vi "Wait Event.vi"(7 "Keep Event Reg (F)":bool, 8 "error in (no error)":errorcluster, 9 "Timeout mS (-1)":i32=-1, 11 "Future in":refnum<class "Future.lvclass">) -> (0 "error out":errorcluster, 1 "Timed Out":bool, 2 "Value":refnum<class>, 3 "Future out":refnum<class "Future.lvclass">)   [LabVIEW 2020, in "Promises.lvlib" / "Future.lvclass"]
uses:
  Future.lvclass
  Future.lvclass/Future.ctl
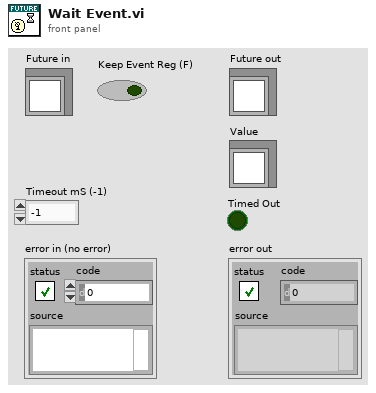
[diagram p1: front panel]
types:
  T1 = typedef "Promises.lvlib/Result State.ctl" = enum16{"Unset", "Error", "Success"}
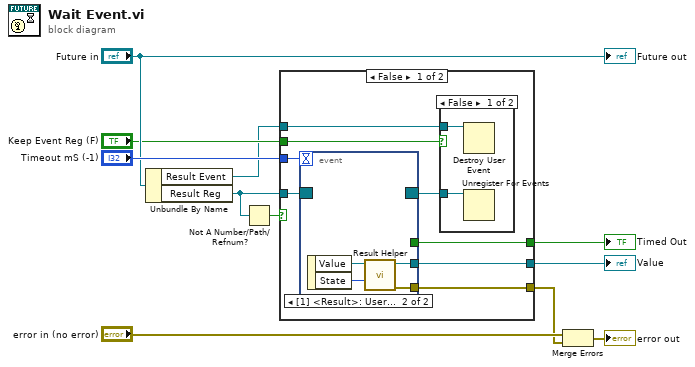
[diagram p0: block diagram]
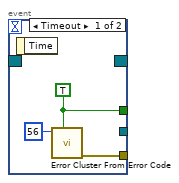
[diagram p2: hidden frame]
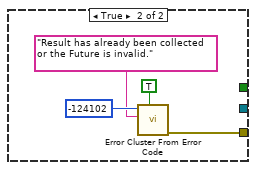
[diagram p4: hidden frame]
diagram:
  n1 = Unbundle By Name("Future in") -> ("Result Event"=w1:refnum<user-event>, "Result Reg"=w5:refnum<event-registration>)
  n2 = Not A Number/Path/Refnum?(number/path/refnum=w5) -> (NaN/Path/Refnum?=w4:bool)
  n3 = case shown="False" w4 {
    tunnel: "Timeout mS (-1)" -> [w19 _]
    tunnel: [w18 _] -> w8
    tunnel: [w17 w32] -> w6
    tunnel: w5 -> [w15 _]
    tunnel: "Keep Event Reg (F)" -> [w14 _]
    tunnel: [w13 _] -> w2
    tunnel: w1 -> [w12 _]
    frame False {
      n4 = event shown="[1] <Result>: User Event" {
        selector: w15 -> [_ _]
        dyn-events: [_ _] -> w16
        timeout: w19 -> [_ _]
        tunnel: [w21 w25] -> w17
        tunnel: [_ w24] -> w18
        tunnel: [w20 _] -> w13
        event Timeout {
          w20 = TRUE ("show call chain? (False)")
          n5 = event-data() -> ()  [unwired: 1 in, 1 out]
          n6 = call <vilib>:"Error Cluster From Error Code.vi"("show call chain? (False)"=w20, "error code (0)"=56) -> ("error out"=w21:errorcluster)  [unwired: 7 in]
        }
        event User Event {
          n7 = event-data() -> ("Value"=w23:refnum<class>, "State"=w26:T1)  [unwired: 1 in]
          n8 = call "Result Helper.vi"("State"=w26, "Value In"=w23) -> ("Error"=w25:errorcluster, "Value"=w24:refnum<class>)  [unwired: 8 in]
        }
      }
      n9 = case shown="False" w14 {
        tunnel: w16 -> [w28 _]
        tunnel: w12 -> [w27 _]
        frame False {
          n10 = Destroy User Event(user event=w27) -> ()  [unwired: 1 in, 1 out]
          n11 = Unregister For Events(event registration refnum=w28) -> ()  [unwired: 1 in, 1 out]
        }
        frame True {
        }
      }
    }
    frame True {
      n12 = call <vilib>:"Error Cluster From Error Code.vi"("show call chain? (False)"=TRUE, "error message (\"\")"="Result has already been collected or the Future is invalid." ("error message (\"\")"), "error code (0)"=-124102) -> ("error out"=w32:errorcluster)  [unwired: 6 in]
    }
  }
  "Value" <- w8
  "Timed Out" <- w2
  n13 = Merge Errors("error in (no error)", w6) -> (→"error out":errorcluster)
  "Future out" <- "Future in"
